vi "Database Check Table Exist.vi"(8 "error in (no error)":errorcluster, 10 "Table Name(\"\")":string, 11 "Database in":refnum<class "DatabaseAPI.lvclass">) -> (0 "error out":errorcluster, 2 "Exit?(True)":bool, 3 "Database out":refnum<class "DatabaseAPI.lvclass">)   [LabVIEW 2015, in "DatabaseAPI.lvclass"]
uses:
  DatabaseAPI.lvclass
  DatabaseAPI.lvclass/DatabaseAPI.ctl
  <vilib>/addons/database/Connection.llb/DB Tools Open Connec (String).vi
  <vilib>/addons/database/Connection.llb/Conn Execute.vi
  <vilib>/addons/database/Recordset.llb/Rec Destroy - Connection.vi
  <vilib>/addons/database/NI_Database_API.lvlib
  <vilib>/addons/database/Recordset.llb/Rec Fetch Recordset Data (R).vi
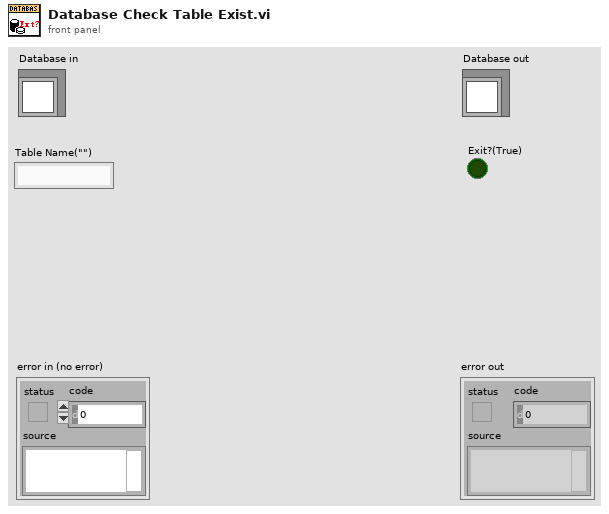
[diagram p1: front panel]
types:
  T1 = typedef "NI_Database_API.lvlib/Conn ObjectReference.ctl" = refnum<k1>
  T2 = typedef "NI_Database_API.lvlib/Rec ObjectReference.ctl" = refnum<k1>
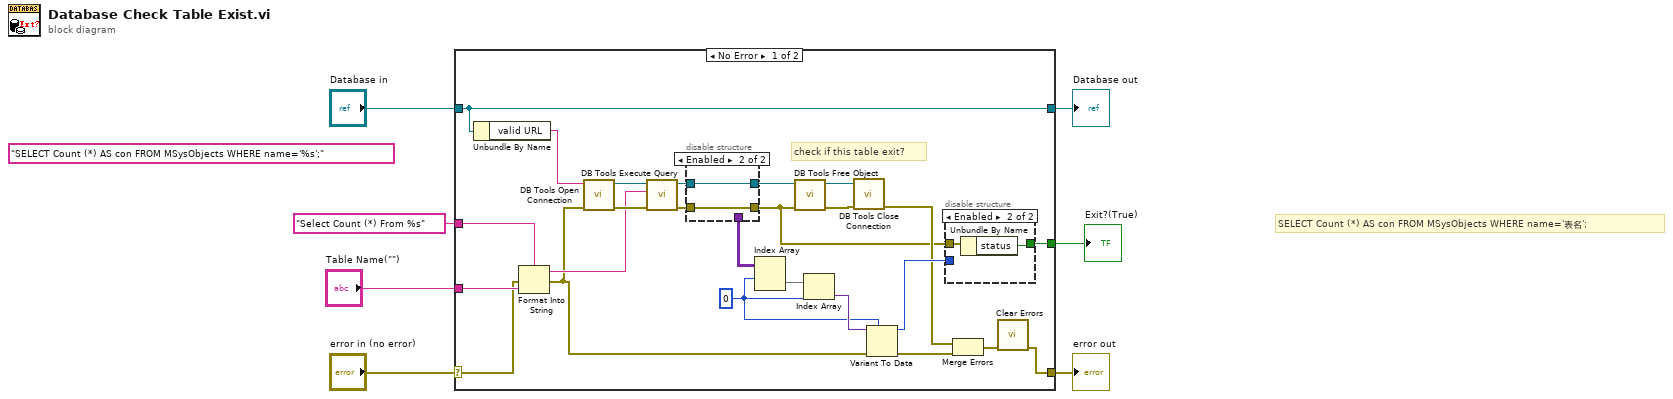
[diagram p0: block diagram]
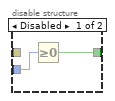
[diagram p2: hidden frame]
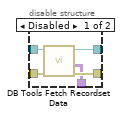
[diagram p3: hidden frame]
diagram:
  (unwired) "SELECT Count (*) AS con FROM MSysObjects WHERE name='%s';" ("format string")
  # "SELECT Count (*) AS con FROM MSysObjects WHERE name='表名';"
  n1 = case shown="No Error" "error in (no error)" {
    selector: "error in (no error)" -> [w24 w45]
    tunnel: [w9 w45] -> w6
    tunnel: [w32 w44] -> w4
    tunnel: "Database in" -> [w32 w44]
    tunnel: "Table Name(\"\")" -> [w25 _]
    tunnel: "Select Count (*) From %s" ("format string") -> [w26 _]
    tunnel: [w14 _] -> w2
    frame No Error {
      w16 = 0 ("index (row)")
      # "check if this table exit?"
      n2 = Unbundle By Name(w32) -> ("valid URL"=w31:string)
      n3 = Format Into String(format string=w26, error in=w24, w25) -> (resulting string=w23:string, error out=w13:errorcluster)  [unwired: 1 in]
      n4 = call-poly <vilib>:"DB Tools Open Connection.vi"("error in (no error)"=w13, "connection information"=w31) -> ("error out"=w29:errorcluster, "connection reference"=w30:T1)  [unwired: 6 in]
      n5 = call-poly <vilib>:"DB Tools Execute Query.vi"("error in (no error)"=w29, "SQL query"=w23, "connection reference"=w30) -> ("error out"=w21:errorcluster, "recordset reference"=w22:T2)  [unwired: 5 in]
      n6 = disable-structure shown="Enabled" {
        disable-tunnel: w22 -> [w41 w43]
        disable-tunnel: w21 -> [w40 w42]
        disable-tunnel: [w39 w43] -> w20
        disable-tunnel: [w38 w42] -> w8
        disable-tunnel: [w37 _] -> w19
        frame Disabled {
          n7 = call-poly <vilib>:"DB Tools Fetch Recordset Data.vi"("error in (no error)"=w40, "recordset reference"=w41) -> ("error out"=w38:errorcluster, "recordset data"=w37:variant[][], "recordset reference out"=w39:T2)  [unwired: 3 in]
        }
        frame Enabled {
        }
      }
      n8 = Index Array(array=w19, index (row)=w16) -> (element=w18:variant[])  [unwired: 1 in]
      n9 = call-poly <vilib>:"DB Tools Free Object.vi"("error in (no error)"=w8, "recordset reference"=w20) -> ("error out"=w27:errorcluster, "connection reference"=w28:T1)  [unwired: 8 in]
      n10 = Index Array(array=w18, index=w16) -> (element=w17:variant)
      n11 = call <vilib>:"DB Tools Close Connection.vi"("error in (no error)"=w27, "connection reference"=w28) -> ("error out"=w11:errorcluster)  [unwired: 5 in]
      n12 = Variant To Data(error in=w13, type=w16, Variant=w17) -> (data=w15:i32, error out=w12:errorcluster)
      n13 = disable-structure shown="Enabled" {
        disable-tunnel: w15 -> [w34 _]
        disable-tunnel: [w33 w35] -> w14
        disable-tunnel: w8 -> [_ w36]
        frame Disabled {
          n14 = Greater Or Equal To 0?(x=w34) -> (x >= 0?=w33:bool)
        }
        frame Enabled {
          n15 = Unbundle By Name(w36) -> ("status"=w35:bool)
        }
      }
      n16 = Merge Errors(w11, w12) -> (w10:errorcluster)
      n17 = call <vilib>:"Clear Errors.vi"("error in (no error)"=w10) -> ("error out"=w9:errorcluster)  [unwired: 5 in, 1 out]
    }
    frame Error {
    }
  }
  "error out" <- w6
  "Database out" <- w4
  "Exit?(True)" <- w2
